vi "OldIntakeTeleop.vi"(8 "CmdCancel":bool, 9 "CmdFeedToShoot":bool, 10 "CmdSpitOut":bool, 11 "CmdIntake":bool) -> ()   [LabVIEW 2023]
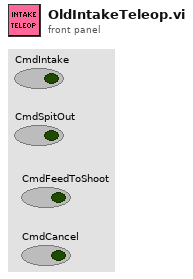
[diagram p1: front panel]
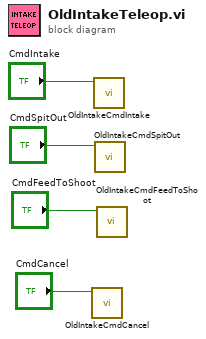
[diagram p0: block diagram]
diagram:
  n1 = call "OldIntakeCmdCancel.vi"("CmdCancel"="CmdCancel") -> ()  [unwired: 11 in]
  n2 = call "OldIntakeCmdIntake.vi"("CmdIntake"="CmdIntake") -> ()  [unwired: 11 in]
  n3 = call "OldIntakeCmdSpitOut.vi"("CmdSpitOut"="CmdSpitOut") -> ()  [unwired: 11 in]
  n4 = call "OldIntakeCmdFeedToShoot.vi"("CmdFeedToShoot"="CmdFeedToShoot") -> ()  [unwired: 11 in]
